vi "ControlSystem.vi"() -> ()   [LabVIEW 2025]
uses:
  <vilib>/OPCUA/controls/NodeId.ctl
  <vilib>/OPCUA/controls/Write Status.ctl
  <vilib>/OPCUA/client/Multiple Write Double.vi
  <vilib>/OPCUA/client/Connect2.vi
  <vilib>/OPCUA/NI OPC UA Client.lvlib
panel:
  out "?":bool
  out "?":bool
  in  "Setpoint [° C]":dbl
  out "Process Value [° C]":dbl format="%#.1g"
  in  "?":bool
  in  "?":enum32{"OPC UA Server", "Controller Settings"}(tab)
  in  "?":string="opc.tcp://LHsPC:49580"
  in  "Setpoint Node":string="ns=2;s=Temperature Setpoint"
  in  "Process Value Node":string="ns=2;s=Temperature Process Value"
  out "Server Status":T1
  in  "Kp":dbl
  in  "Ti":dbl
  in  "Ts":dbl
  out "Control signal [V]":dbl format="%#_2g"
  out "Error [° C]":dbl
  in  "Tuning Mode":bool
  out "?":dynamicdata(graph)
  # "Air Heater Operation"
  # "Alarm Status"
  # "Server URL"
  # "PI Parameters"
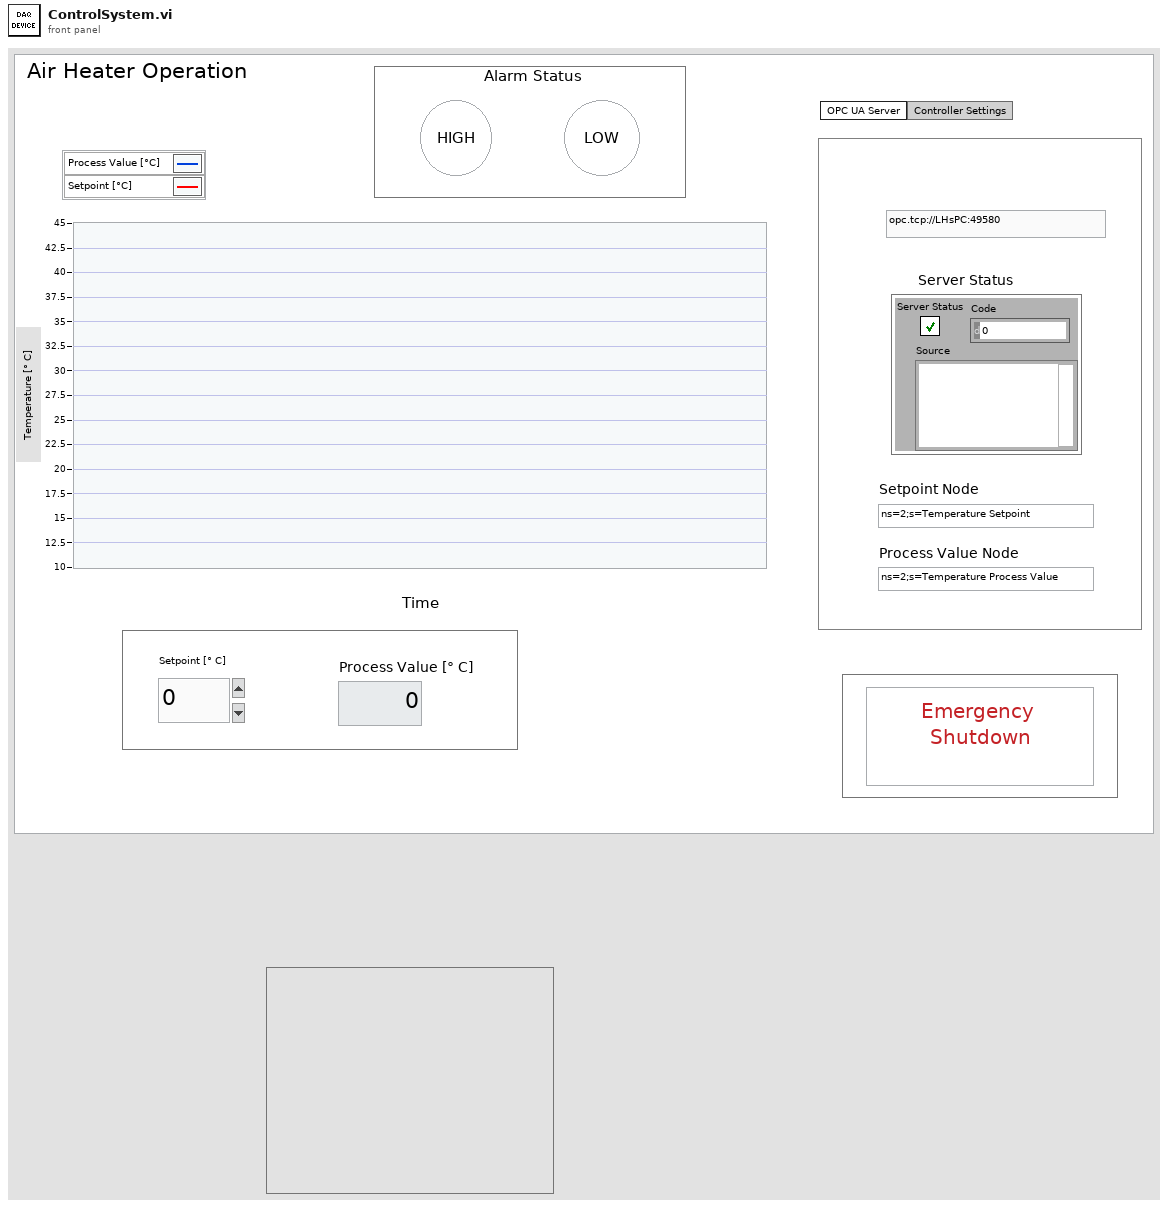
[diagram p1: front panel]
types:
  T1 = cluster{"Server Status":bool, "Code":i32, "Source":string}
  T2 = typedef "OPC UA Client Refnum.ctl" = refnum<k21>
  T3 = typedef "NodeId.ctl" = string
  T4 = typedef "Write Status.ctl" = u32
  T5 = cluster{"node ID":T3, "value":dbl, "timestamp (current time)":timestamp, "node status":T4}
  T6 = enum8{"Enabled", "Disabled", "Disabled and Grayed Out"}
  T7 = cluster{"node ID":T3, "value":dbl, "timestamp (current time)":timestamp, "node status":T4}[]
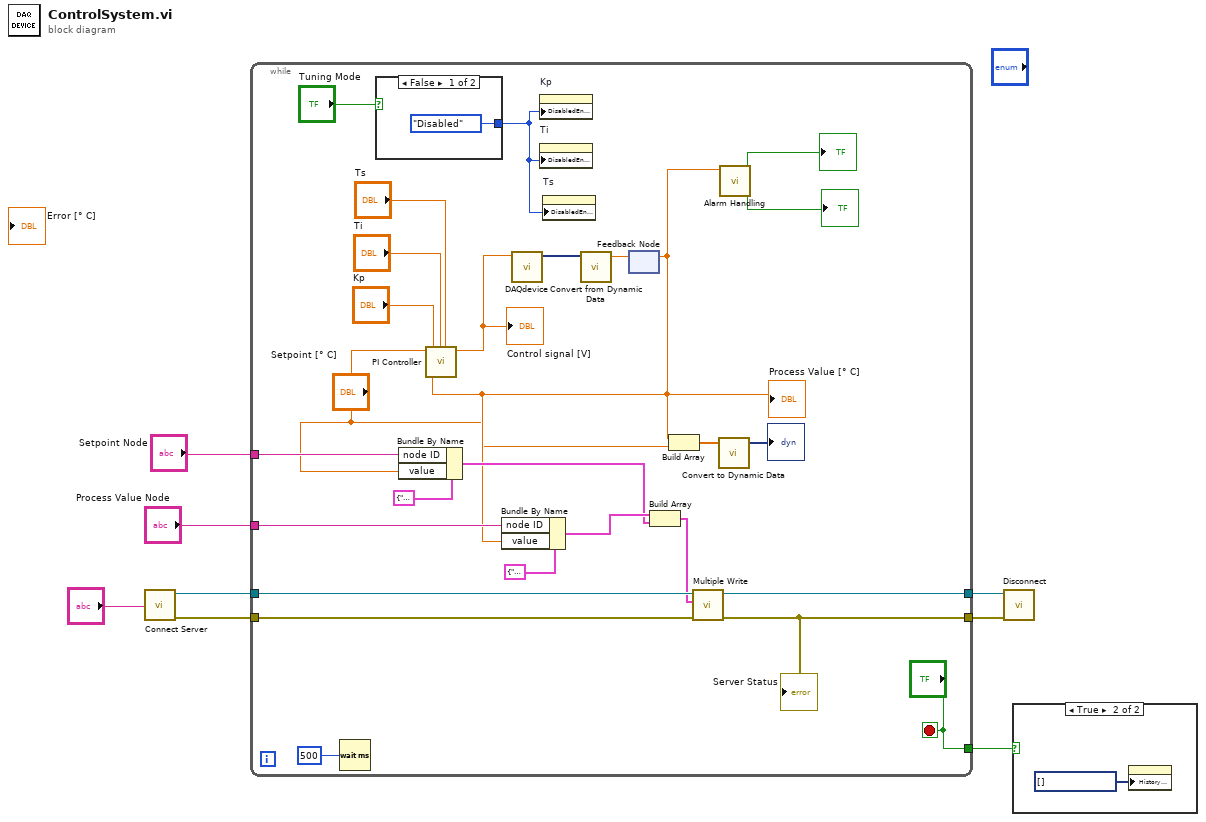
[diagram p0: block diagram]
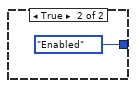
[diagram p3: hidden frame]
diagram:
  n1 = call-poly <vilib>:"Connect Server.vi"("server endpoint URL"="?") -> ("error out"=w3:errorcluster, "OPC UA client refnum out"=w7:T2)  [unwired: 8 in, 1 out]
  n2 = while {
    tunnel: ["?"] -> w1
    tunnel: [w33] -> w8
    tunnel: w7 -> [w32]
    tunnel: "Process Value Node" -> [w30]
    tunnel: "Setpoint Node" -> [w29]
    tunnel: w3 -> [w24]
    tunnel: [w23] -> w2
    stop <- "?" stop-if-true
    n3 = Wait (ms)(milliseconds to wait=u32 500 ("millisecond timer value")) -> ()  [unwired: 1 out]
    n4 = case shown="False" "Tuning Mode" {
      tunnel: [T6."Disabled" ("Disabled") T6."Enabled" ("Disabled")] -> w10
      frame False {
      }
      frame True {
      }
    }
    n5 = Bundle By Name "Bundle By Name"(cluster=T5 {"node ID"="", "value"=0.0, "timestamp (current time)"=timestamp(0 s since 1904-01-01), "node status"=0} ("request"), "node ID"=w29, "value"="Setpoint [° C]") -> (w26:T5)
    n6 = property on="Kp" class="DigNum (strict)"("DisabledEnum"=w10) -> ()  [unwired: 2 in, 2 out]
    n7 = property on="Ti" class="DigNum (strict)"("DisabledEnum"=w10) -> ()  [unwired: 2 in, 2 out]
    n8 = property on="Ts" class="DigNum (strict)"("DisabledEnum"=w10) -> ()  [unwired: 2 in, 2 out]
    n9 = feedback #1() -> (w12:dbl)  [unwired: 1 in]
    "Process Value [° C]" <- w12
    n10 = call "PI Controller.vi"("Ti"="Ti", "Ts"="Ts", "Kp"="Kp", "yk"=w12, "rk"="Setpoint [° C]") -> ("Control signal"=w15:dbl)  [unwired: 6 in]
    "Control signal [V]" <- w15
    n11 = Bundle By Name "Bundle By Name"(cluster=T5 {"node ID"="", "value"=0.0, "timestamp (current time)"=timestamp(0 s since 1904-01-01), "node status"=0} ("request"), "node ID"=w30, "value"=w12) -> (w27:T5)
    n12 = call "DAQdevice.vi"("data in"=w15) -> ("data out"=w14:dynamicdata)  [unwired: 10 in]
    n13 = call "Convert from Dynamic Data"("Dynamic Data Type"=w14) -> ("Scalar"=w13:dbl)  [unwired: 3 in]
    n14 = feedback-in #1(w13) -> ()
    n15 = Build Array "Build Array"(w27, w26) -> (w25:T7)
    n16 = Build Array "Build Array"(w12, "Setpoint [° C]") -> (w22:dbl[])
    n17 = call-poly <vilib>:"Multiple Write.vi"("error in (no error)"=w24, "requests"=w25, "OPC UA client refnum in"=w32) -> ("error out"=w23:errorcluster, "OPC UA client refnum out"=w33:T2)  [unwired: 5 in, 2 out]
    "Server Status" <- w23
    n18 = call "Convert to Dynamic Data"("Array"=w22) -> ("Dynamic Data Type"=→"?":dynamicdata)  [unwired: 3 in]
    n19 = call "Alarm Handling.vi"("yk"=w12) -> ("Boolean"=→"?":bool, "Boolean 2"=→"?":bool)  [unwired: 9 in]
  }
  n20 = call <vilib>:"Disconnect.vi"("error in (no error)"=w2, "OPC UA client refnum in"=w8) -> ()  [unwired: 9 in, 1 out]
  n21 = case shown="True" w1 {
    frame False {
    }
    frame True {
      n22 = property class="WFChart (strict)"("History Data"=dynamicdata[] []) -> ()  [unwired: 2 in, 2 out]
    }
  }
